vi "Sol 3 Func Gen Sound Python Complete.vi"() -> ()   [LabVIEW 2025]
uses:
  <vilib>/sound2/lvsound2.llb/Sound Data Format.ctl
  <vilib>/Analysis/2dsp.llb/Real FFT.vi
  <vilib>/sound2/lvsound2.llb/Sound Output Write (DBL Single).vi
  <vilib>/measure/NI_MABase.lvlib
  <vilib>/Analysis/NI_AALPro.lvlib
panel:
  out "Signal":dbl[](graph)
  in  "length pts":dbl=30000.0
  out "Waveform Graph":waveform(dbl)(graph)={"t0"=timestamp(0 s since 1904-01-01), "dt"=0.001, "Y"=array[1000 elements]}
  in  "dt":dbl=0.0001
  in  "Freq Stop":dbl=500.0
  in  "Freq Start":dbl=100.0
  in  "Amp":dbl=1.0
  in  "Amplitude":dbl=2.0
  in  "Frequency":dbl=10.0
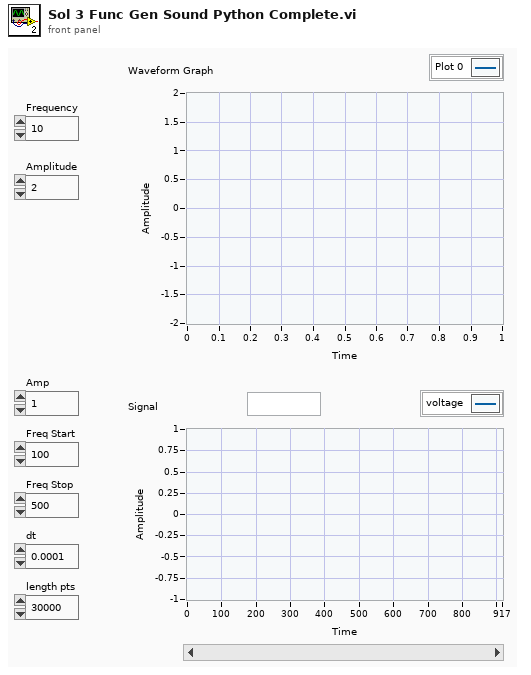
[diagram p1: front panel]
types:
  T1 = enum16{"Sine Wave", "Triangle Wave", "Square Wave", "Sawtooth Wave"}
  T2 = typedef "Sound Data Format.ctl" = cluster{"sample rate (S/s)":dbl, "number of channels":i32, "bits per sample":i32}
  T3 = typedef "Sound Output Task ID.ctl" = u32
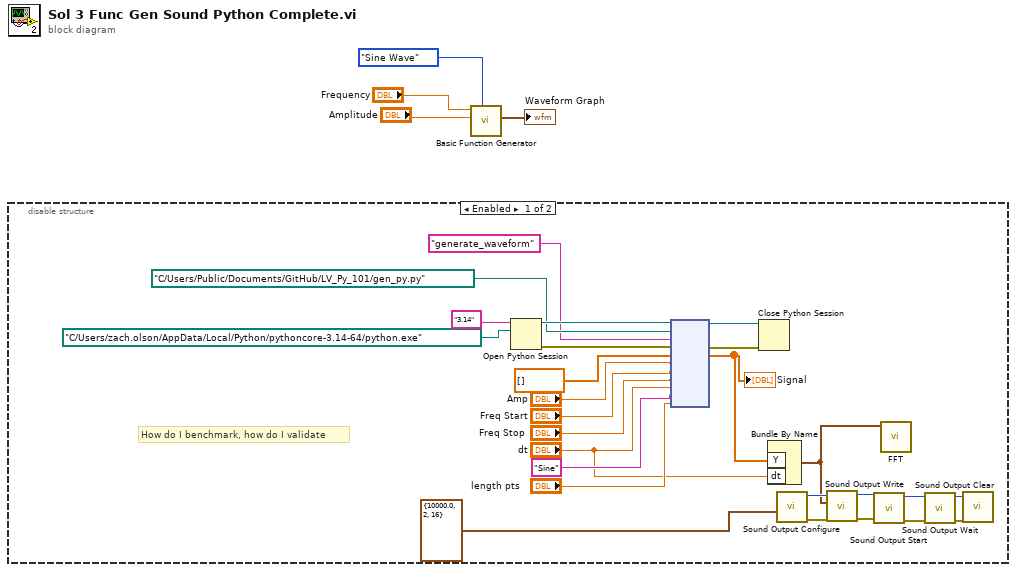
[diagram p0: block diagram]
diagram:
  n1 = disable-structure shown="Enabled" {
    frame Enabled {
      # "How do I benchmark, how do I validate"
      n2 = Open Python Session(python version="3.14" ("Python version"), python path=path "C:/Users/zach.olson/AppData/Local/Python/pythoncore-3.14-64/python.exe" ("Python path")) -> (session out=w28:refnum<k35>, error out=w27:errorcluster)  [unwired: 1 in]
      n3 = node(w28, path "C:/Users/Public/Documents/GitHub/LV_Py_101/gen_py.py" ("module path"), "generate_waveform" ("function name"), w27, dbl[] [], "Amp", "Freq Start", "Freq Stop", "dt", "Sine", "length pts") -> (w26:refnum<k35>, w25:errorcluster, w8:dbl[])  [unwired: 6 in, 2 out]
      "Signal" <- w8
      n4 = Close Python Session(session in=w26, error in=w25) -> ()  [unwired: 1 out]
      n5 = Bundle By Name("Y"=w8, "dt"="dt") -> (w5:waveform(dbl))  [unwired: 1 in]
      n6 = call <vilib>:"Sound Output Configure.vi"("sound format"=T2 {"sample rate (S/s)"=10000.0, "number of channels"=2, "bits per sample"=16}) -> ("error out"=w9:errorcluster, "task ID"=w10:T3)  [unwired: 9 in]
      n7 = call-poly <vilib>:"Sound Output Write.vi"("error in (no error)"=w9, "data"=w5, "task ID"=w10) -> ("error out"=w11:errorcluster, "task ID out"=w12:T3)  [unwired: 7 in]
      n8 = call <vilib>:"Sound Output Start.vi"("error in (no error)"=w11, "task ID"=w12) -> ("error out"=w13:errorcluster, "task ID out"=w14:T3)  [unwired: 8 in]
      n9 = call-poly <vilib>:"FFT.vi"("X"=w5) -> ()  [unwired: 9 in, 2 out]
      n10 = call <vilib>:"Sound Output Wait.vi"("error in (no error)"=w13, "task ID"=w14) -> ("error out"=w16:errorcluster, "task ID out"=w15:T3)  [unwired: 8 in]
      n11 = call <vilib>:"Sound Output Clear.vi"("error in (no error)"=w16, "task ID"=w15) -> ()  [unwired: 9 in, 1 out]
    }
    frame Disabled {
    }
  }
  n12 = call <vilib>:"Basic Function Generator.vi"("signal type"=T1."Sine Wave", "amplitude"="Amplitude", "frequency"="Frequency") -> ("signal out"=→"Waveform Graph":waveform(dbl))  [unwired: 6 in, 2 out]
